vi "Extract Digits.vi"(11 "Message":u8[](array[numeric]) format="%.0x") -> (2 "Valid":bool, 3 "DMM digits":dbl)   [LabVIEW 2015, in "VC940.lvlib"]
uses:
  VC940.lvlib
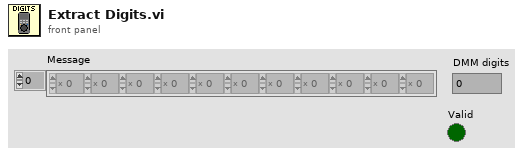
[diagram p1: front panel]
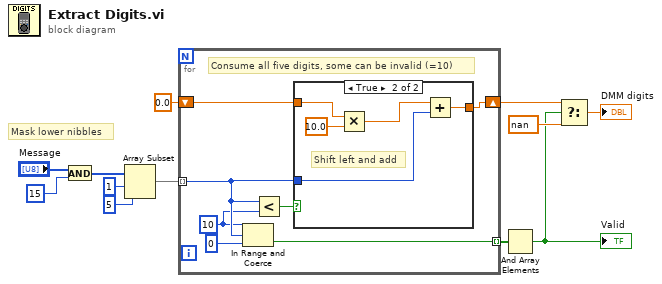
[diagram p0: block diagram]
diagram:
  # "Mask lower nibbles"
  n1 = And(x="Message", y=u8 15) -> (x .and. y?=w4:u8[])
  n2 = Array Subset(array=w4, index=1, length=5) -> (w7:u8[])
  n3 = for {
    tunnel: w7 -> [w16] mode=indexing
    shift-right: [w19] -> w10
    shift-left: 0.0 -> [w13]
    tunnel: [w17] -> w9 mode=indexing
    w15 = 10 ("upper limit")
    # "Consume all five digits, some can be invalid (=10)"
    n4 = In Range and Coerce(upper limit=w15, x=w16, lower limit=0) -> (In Range?=w17:bool)  [unwired: 1 out]
    n5 = Less?(x=w16, y=w15) -> (x < y?=w14:bool)
    n6 = case shown="True" w14 {
      tunnel: w13 -> [w20 w22]
      tunnel: [w20 w25] -> w19
      tunnel: w16 -> [_ w24]
      frame False {
        # "Ignore digit"
      }
      frame True {
        # "Shift left and add"
        n7 = Multiply(x=w22, y=10.0) -> (x*y=w21:dbl)
        n8 = Add(x=w21, y=w24) -> (x+y=w25:dbl)
      }
    }
  }
  n9 = And Array Elements(Boolean array=w9) -> (logical AND=w2:bool)
  "Valid" <- w2
  n10 = Select(t=w10, s=w2, f=nan) -> (s? t:f=→"DMM digits":dbl)
